vi "SERIAL_VerifyChecksum.vi"(1 "ExpectedFullPacketLength":i32, 2 "Packet\n\n\n\n\n\n\n\n\n\n\n\n\n\nPacketContent":string) -> (0 "Valid Checksum":bool)   [LabVIEW 2014, in "navX-MXP IMU.lvlib"]
uses:
  navX-MXP IMU.lvlib
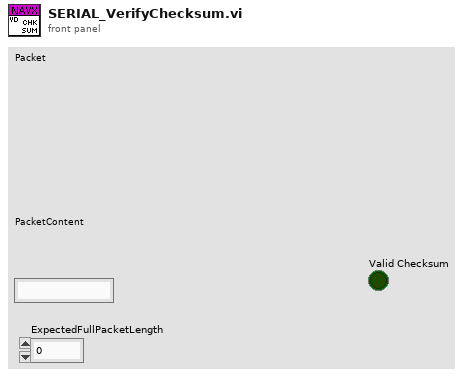
[diagram p1: front panel]
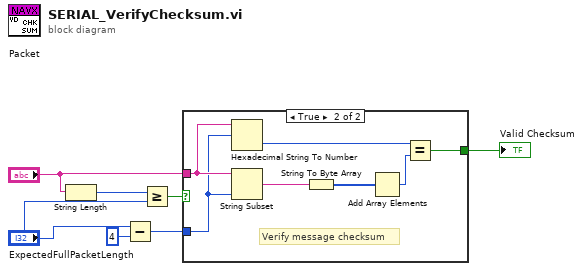
[diagram p0: block diagram]
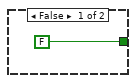
[diagram p2: hidden frame]
diagram:
  n1 = String Length(string="Packet\n\n\n\n\n\n\n\n\n\n\n\n\n\nPacketContent") -> (length=w3:i32)
  n2 = Subtract(x="ExpectedFullPacketLength", y=4) -> (x-y=w5:i32)
  n3 = Greater Or Equal?(x=w3, y="ExpectedFullPacketLength") -> (x >= y?=w1:bool)
  n4 = case shown="True" w1 {
    tunnel: "Packet\n\n\n\n\n\n\n\n\n\n\n\n\n\nPacketContent" -> [_ w13]
    tunnel: w5 -> [_ w9]
    tunnel: [FALSE w10] -> w4
    frame False {
    }
    frame True {
      # "Verify message checksum"
      n5 = Hexadecimal String To Number(string=w13, offset=w9) -> (number=w11:u32)  [unwired: 1 in, 1 out]
      n6 = String Subset(string=w13, length (rest)=w9) -> (substring=w14:string)  [unwired: 1 in]
      n7 = String To Byte Array(string=w14) -> (unsigned byte array=w15:u8[])
      n8 = Add Array Elements(numeric array=w15) -> (sum=w12:u8)
      n9 = Equal?(x=w11, y=w12) -> (x = y?=w10:bool)
    }
  }
  "Valid Checksum" <- w4
